vi "WD_SWA_substract_last.vi"(8 "error in (no error)":errorcluster, 11 "DBLink":string="Driver={ODBC Driver 17 for SQL Server};Server=localhost\\SQLEXPRESS;Database=ZDX201;UID=labview;PWD=Dsa@54137926") -> (0 "error out":errorcluster, 1 "站點總數":i32, 2 "當前料數":i32, 3 "計算用 array":cluster{"條碼A":string, "條碼B":string}[](array[cluster]), 4 "取出element":cluster{"條碼A":string, "條碼B":string}, 5 "顯示用array":cluster{"條碼A":string, "條碼B":string}[](array[cluster]))   [LabVIEW 2019]
panel:
  out "x-y":i32
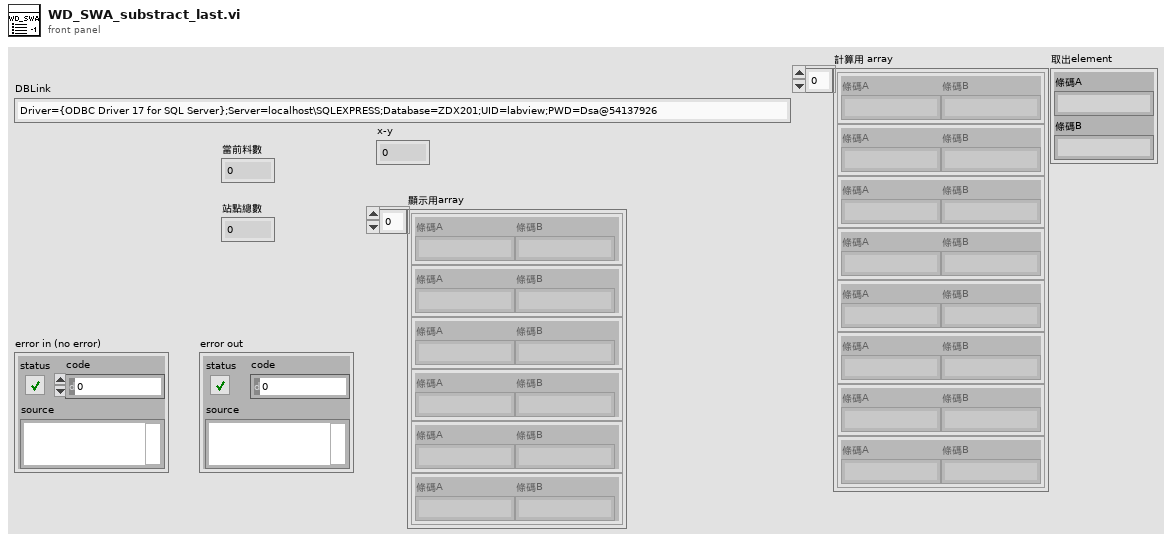
[diagram p1: front panel]
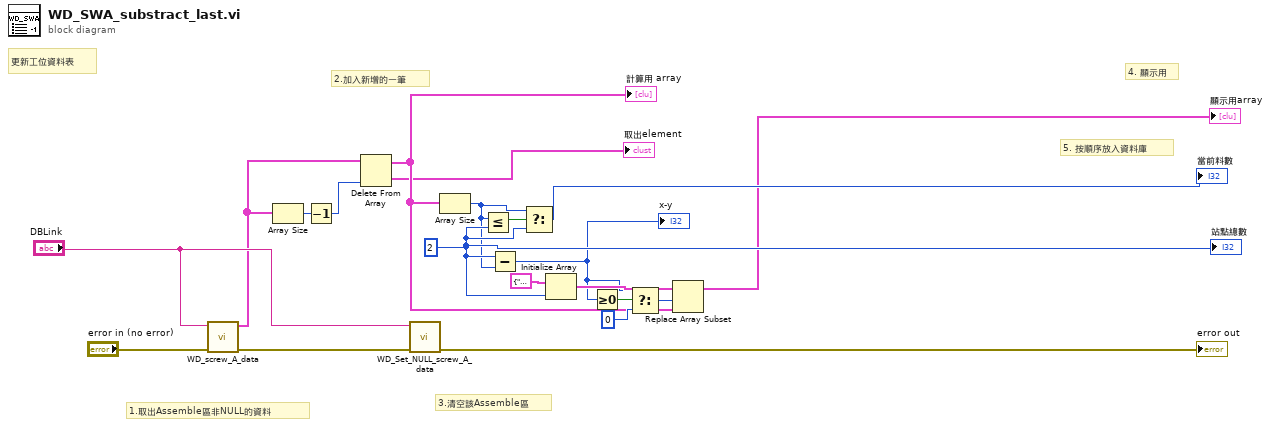
[diagram p0: block diagram]
diagram:
  w17 = 2
  # "5. 按順序放入資料庫"
  # "4. 顯示用"
  # "3.清空該Assemble區"
  # "2.加入新增的一筆"
  # "1.取出Assemble區非NULL的資料"
  # "更新工位資料表"
  n1 = call "WD_screw_A_data.vi"("error in (no error)"="error in (no error)", "DBlink"="DBLink") -> ("error out"=w7:errorcluster, "鎖A備料"=w1:cluster{"條碼A":string, "條碼B":string}[])  [unwired: 6 in, 2 out]
  n2 = Array Size(array=w1) -> (size(s)=w5:i32)
  n3 = Decrement(x=w5) -> (x-1=w4:i32)
  n4 = Delete From Array(array=w1, index=w4) -> (deleted portion=→"取出element":cluster{"條碼A":string, "條碼B":string}, array with subset deleted=w3:cluster{"條碼A":string, "條碼B":string}[])  [unwired: 1 in]
  "計算用 array" <- w3
  n5 = call "WD_Set_NULL_screw_A_data.vi"("error in (no error)"=w7, "DBlink"="DBLink") -> ("error out"=→"error out":errorcluster)  [unwired: 8 in, 1 out]
  n6 = Array Size(array=w3) -> (size(s)=w16:i32)
  n7 = Less Or Equal?(x=w16, y=w17) -> (x <= y?=w19:bool)
  n8 = Subtract(x=w17, y=w16) -> (x-y=w11:i32)
  "x-y" <- w11
  n9 = Select(t=w16, s=w19, f=w17) -> (s? t:f=→"當前料數":i32)
  n10 = Initialize Array(cluster{"條碼A":string, "條碼B":string} {"條碼A"="NULL", "條碼B"="NULL"} ("New data"), w17) -> (w18:cluster{"條碼A":string, "條碼B":string}[])
  n11 = Greater Or Equal To 0?(x=w11) -> (x >= 0?=w13:bool)
  n12 = Select(t=w11, s=w13, f=i16 0) -> (s? t:f=w10:i32)
  n13 = Replace Array Subset(array=w18, new element=w3, index=w10) -> (→"顯示用array":cluster{"條碼A":string, "條碼B":string}[])
  "站點總數" <- w17
